vi "main.vi"() -> ()   [LabVIEW 2021]
panel:
  out "Boolean":bool caption="Now you can use the local router!"
  out "IP":string
  # "Local IP"
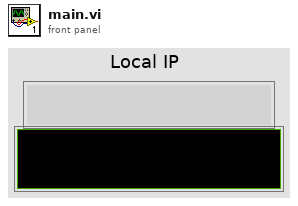
[diagram p1: front panel]
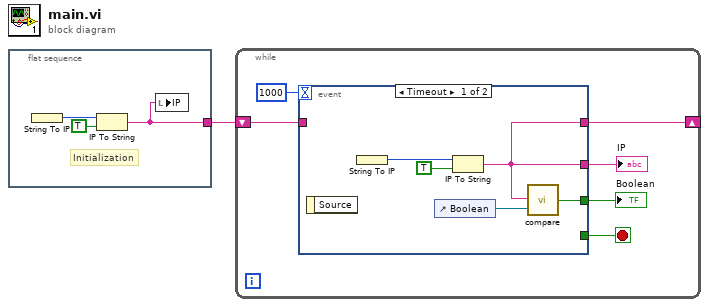
[diagram p0: block diagram]
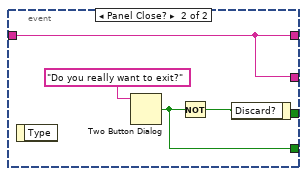
[diagram p2: hidden frame]
diagram:
  n1 = flat-sequence {
    tunnel: [w2] -> w1
    frame #0 {
      # "Initialization"
      n2 = String To IP() -> (0:w3:u32)  [unwired: 1 in]
      n3 = IP To String(1:TRUE ("dot notation? (F)"), 2:w3) -> (0:w2:string)
      n4 = local write "IP"(w2) -> ()
    }
  }
  n5 = while {
    shift-right: [w7] -> _
    shift-left: w1 -> [w8]
    stop <- w9 stop-if-true
    n6 = event shown="[0] Timeout" {
      selector: _ -> [_ _]
      dyn-events: _ -> [_ _]
      timeout: 1000 -> [_ _]
      tunnel: [w11 w16] -> w6
      tunnel: [_ w17] -> w9
      tunnel: w8 -> [_ w16]
      tunnel: [w11 w16] -> w7
      tunnel: [w13 _] -> w5
      event Timeout {
        n7 = event-data() -> ()  [unwired: 1 in, 1 out]
        n8 = String To IP() -> (0:w15:u32)  [unwired: 1 in]
        n9 = control-ref of="Boolean"() -> (w12:refnum<vi>)
        n10 = IP To String(1:TRUE ("dot notation? (F)"), 2:w15) -> (0:w11:string)
        n11 = call "compare.vi"("isOk?"=w12, "IP"=w11) -> ("isOk?"=w13:bool)
      }
      event Panel Close? {
        n12 = event-data() -> ()  [unwired: 1 in, 1 out]
        n13 = Two Button Dialog(message="Do you really want to exit?") -> (T button?=w17:bool)  [unwired: 2 in]
        n14 = Not(x=w17) -> (.not. x?=w18:bool)
        n15 = event-data("Discard?"=w18) -> ()  [unwired: 1 in, 1 out]
      }
    }
    "IP" <- w6
    "Boolean" <- w5
  }
